vi "test-diff-drive-kine-constraint.vi"(8 "error in (no error)":errorcluster) -> (0 "error out 2":errorcluster, 3 "Test Passed":bool)   [LabVIEW 2019]
uses:
  <vilib>/Rock Robotics/WPI/ThirdParty/JAS_Junk/TrajLib/POSE2D.ctl
  <vilib>/Rock Robotics/WPI/ThirdParty/JAS_Junk/TrajLib/TRANSLATION2D.ctl
  <vilib>/Rock Robotics/WPI/ThirdParty/JAS_Junk/TrajLib/ROTATION2D.ctl
  <vilib>/Rock Robotics/SystemInterfaces/NetworkCommunication/NetComm_UsageReport_report.vi
  <vilib>/Rock Robotics/WPI/ThirdParty/JAS_Junk/TrajLib/DiffDriveKinematicsConstraint_New.vi
  <vilib>/Rock Robotics/WPI/ThirdParty/JAS_Junk/TrajLib/Util_LibraryGlobals.vi
  <vilib>/Rock Robotics/WPI/ThirdParty/JAS_Junk/TrajLib/Trajectory_Library.lvlib
panel:
  out "Accel Exceeded":bool
  out "Acceleration":dbl[][](graph)
  out "Velocity":dbl[][](graph)
  out "Max Accel":dbl
  out "Max Ya":dbl
  out "max Xx":dbl
  in  "Feet/Sec":dbl=12.0 format="%#_13g"
  in  "Feet Per Sec^2":dbl=12.0 format="%#_13g"
  out "Max Speed":dbl
  out "Max Y vel":dbl
  out "max X vel":dbl
  out "XY Graph":cluster{dbl[], dbl[]}[](graph)
  out "Waypoints":T1[](array[typedef]) {"ROTATION"."SIN" format="%13.4f"; "ROTATION"."COS" format="%13.4f"; "ROTATION"."VALUE" format="%13.4f"; "TRANSLATION"."Y" format="%14.3f"; "TRANSLATION"."X" format="%14.3f"}
  out "TotalTImeSecs":dbl
  out "Speed Exceeded":bool
  out "error out":errorcluster
  # "9.1"
  # "5.7"
  # "9.55"
  # "6.59"
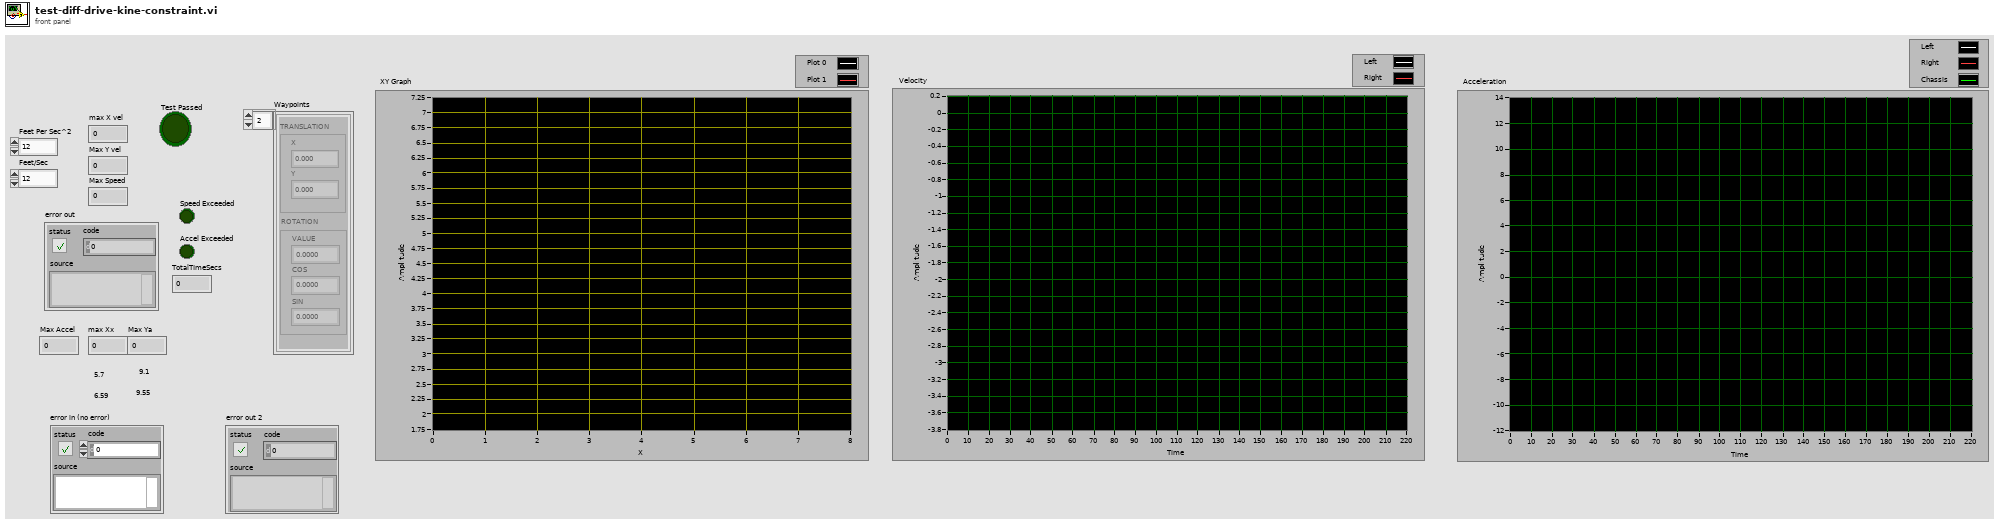
[diagram p1: front panel]
types:
  T1 = typedef "Trajectory_Library.lvlib/POSE2D.ctl" = cluster{"TRANSLATION":T2, "ROTATION":T3}
  T2 = typedef "Trajectory_Library.lvlib/TRANSLATION2D.ctl" = cluster{"X":dbl, "Y":dbl}
  T3 = typedef "Trajectory_Library.lvlib/ROTATION2D.ctl" = cluster{"VALUE":dbl, "COS":dbl, "SIN":dbl}
  T4 = typedef "Trajectory_Library.lvlib/TRAJ_CONFIG.ctl" = cluster{"MaxVelocity":dbl, "Max Acceleration":dbl, "StartVelocity":dbl, "End Velocity":dbl, "Reversed":bool, "DiffDrKineConstntDefined":bool, "CentAcellConstntDefined":bool, "DiffDrVoltConstntDefined":bool, "DIFF_DRIVE_KINE_CONSTRAINT":T5, "CENTRIPETAL_ACCEL_CONSTRAINT":T7, "SwerveDrKineConstntDefined":bool, "SWERVE_DRIVE_KINE_CONSTRAINT":T8, "DIFF_DRIVE_VOLTAGE_CONSTRAINT":T11, "MECANUM_DRIVE_KINE_CONSTRAINT":T13, "MecanumDrKineConstntDefined":bool}
  T5 = typedef "Trajectory_Library.lvlib/TRAJ_CONSTRAINT_DIIF_DRIVE_KINEMATICS.ctl" = cluster{"Max Speed (M/S)":dbl, "DIFF_DRIVE_KINEMATICS":T6, "Max Accel (M/S2)":dbl}
  T6 = typedef "Trajectory_Library.lvlib/DIFF_DRIVE_KINEMATICS.ctl" = cluster{"TrackWidth_Meters":dbl}
  T7 = typedef "Trajectory_Library.lvlib/TRAJ_CONSTRAINT_CENTRIPETAL_ACCEL.ctl" = cluster{"Max Cent Accel":dbl}
  T8 = typedef "Trajectory_Library.lvlib/TRAJ_CONSTRAINT_SWERVE_DRIVE_KINEMATICS.ctl" = cluster{"Max Speed (M/S)":dbl, "SwerveKinematics":T9}
  T9 = typedef "Trajectory_Library.lvlib/SWERVE_DRIVE_KINEMATICS.ctl" = cluster{"NumModules":i32, "InverseKinematics":T10, "ForwardKinematics":T10, "Modules":T2[], "PrevCoR":T2}
  T10 = typedef "NI_Matrix.lvlib/RealMatrix.ctl" = dbl[][]
  T11 = typedef "Trajectory_Library.lvlib/TRAJ_CONSTRAINT_DIIF_DRIVE_VOLTAGE.ctl" = cluster{"Max Voltage":dbl, "DIFF_DRIVE_KINEMATICS":T6, "SIMPLE_MOTOR_FF":T12}
  T12 = typedef "Trajectory_Library.lvlib/SIMPLE_MOTOR_FF.ctl" = cluster{"Ks":dbl, "Kv":dbl, "Ka":dbl}
  T13 = typedef "Trajectory_Library.lvlib/TRAJ_CONSTRAINT_MECA_DRIVE_KINEMATICS.ctl" = cluster{"Max Speed (M/S)":dbl, "MECA_DRIVE_KINEMATICS":T14}
  T14 = typedef "Trajectory_Library.lvlib/MECA_DRIVE_KINEMATICS.ctl" = cluster{"FrontLeft":T2, "FrontRight":T2, "RearLeft":T2, "RearRight":T2, "InverseKinematics":T10, "ForwardKinematics":T10, "PrevCoR":T2}
  T15 = typedef "Trajectory_Library.lvlib/TRAJECTORY.ctl" = cluster{"TotalTImeSecs":dbl, "States":T16[]}
  T16 = typedef "Trajectory_Library.lvlib/TRAJ_STATE.ctl" = cluster{"TimeSeconds":dbl, "Velocity":dbl, "Acceleration":dbl, "POSE":T1, "Curvature":dbl}
  T17 = typedef "Trajectory_Library.lvlib/CHASSIS_SPEEDS.ctl" = cluster{"vX":dbl, "vY":dbl, "vOmega":dbl}
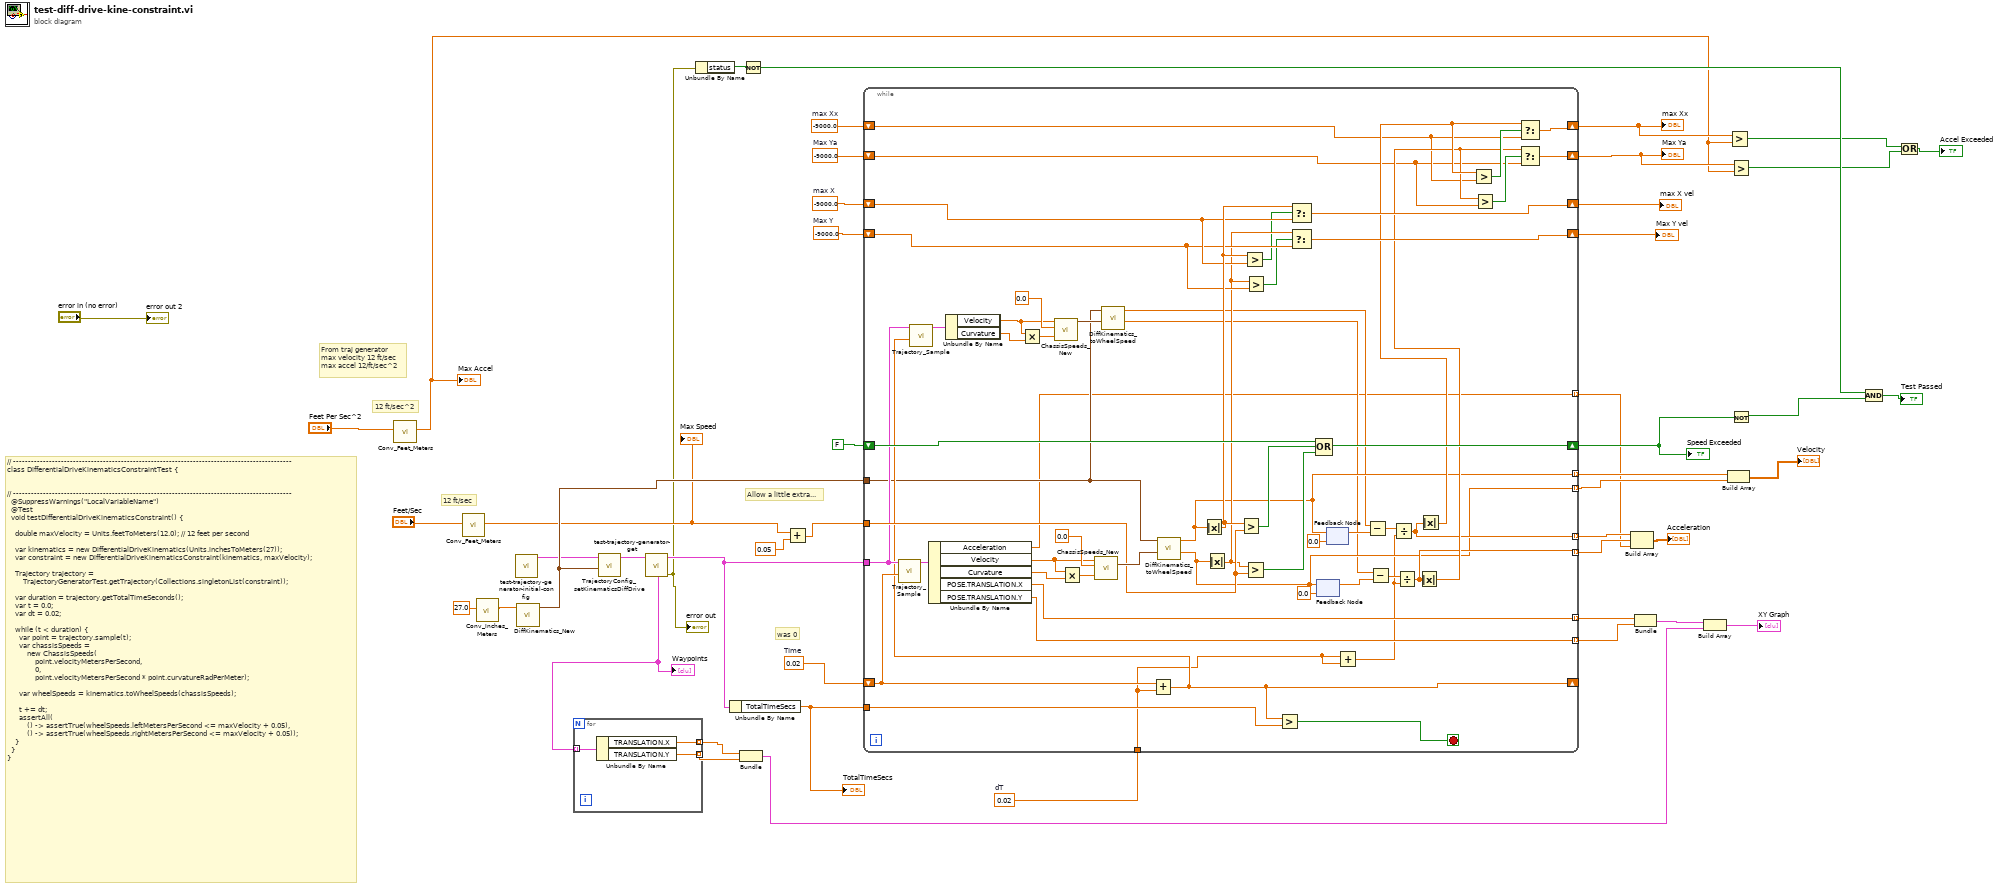
[diagram p0: block diagram]
diagram:
  w17 = -9000.0  # max Xx
  w18 = -9000.0  # Max Ya
  w27 = -9000.0  # max X
  w28 = -9000.0  # Max Y
  w43 = 0.02  # dT
  w45 = 0.02  # TIme
  # "was 0"
  # "Allow a little extra..."
  # "12 ft/sec^2"
  # "From traj generator\nmax velocity 12 ft/sec\nmax accel 12/ft/sec^2"
  # "12 ft/sec"
  # "// ---------------------------------------------------------------------------------------------\nclass DifferentialDriveKinematicsConstraintTest {\n\n\n// ---------------------------------------------------------------------------------------------\n  @SuppressWarnings(\"LocalVariableName\")\n  @Test\n  void testDifferentialDriveKinematicsConstraint() {\n\n    double maxVelocity = Units.feetToMeters(12.0); // 12 feet per second\n\n    var kinematics = new DifferentialDriveKinematics(Units.inchesToMeters(27));\n    var constraint = new DifferentialDriveKinematicsConstraint(kinematics, maxVelocity);\n\n    Trajectory trajectory =\n        TrajectoryGeneratorTest.getTrajectory(Collections.singletonList(constraint));\n\n    var duration = trajectory.getTotalTimeSeconds();\n    var t = 0.0;\n    var dt = 0.02;\n\n    while (t < duration) {\n      var point = trajectory.sample(t);\n      var chassisSpeeds =\n          new ChassisSpeeds(\n              point.velocityMetersPerSecond,\n              0,\n              point.velocityMetersPerSecond * point.curvatureRadPerMeter);\n\n      var wheelSpeeds = kinematics.toWheelSpeeds(chassisSpeeds);\n\n      t += dt;\n      assertAll(\n          () -> assertTrue(wheelSpeeds.leftMetersPerSecond <= maxVelocity + 0.05),\n          () -> assertTrue(wheelSpeeds.rightMetersPerSecond <= maxVelocity + 0.05));\n    }\n  }\n}"
  n1 = call <vilib>:"Conv_Feet_Meters.vi"("Feet"="Feet Per Sec^2") -> ("Meters"=w4:dbl)  [unwired: 10 in]
  "Max Accel" <- w4
  n2 = call <vilib>:"Conv_Feet_Meters.vi"("Feet"="Feet/Sec") -> ("Meters"=w39:dbl)  [unwired: 10 in]
  "Max Speed" <- w39
  n3 = call <vilib>:"Conv_Inches_Meters.vi"("INCH"=27.0) -> ("Meters"=w49:dbl)  [unwired: 10 in]
  n4 = call "test-trajectory-generator-initial-config.vi"() -> ("traj_config"=w2:T4)  [unwired: 11 in]
  n5 = call <vilib>:"DiffKinematics_New.vi"("TrackWidth_Meters"=w49) -> ("DIFF_DRIVE_KINEMATICS"=w41:T6)  [unwired: 10 in]
  n6 = call <vilib>:"TrajectoryConfig_setKinematicsDiffDrive.vi"("DIFF_DRIVE_KINEMATICS"=w41, "inTRAJECTORY_CONFIG"=w2) -> ("outTRAJECTORY_CONFIG"=w3:T4)  [unwired: 9 in]
  n7 = call "test-trajectory-generator-get.vi"("traj_config"=w3) -> ("error out"=w21:errorcluster, "TRAJECTORY"=w42:T15, "Waypoints"=w36:T1[])  [unwired: 8 in]
  "error out" <- w21
  "Waypoints" <- w36
  n8 = for {
    tunnel: w36 -> [w52] mode=indexing
    tunnel: [w51] -> w35 mode=indexing
    tunnel: [w50] -> w34 mode=indexing
    n9 = Unbundle By Name(w52) -> ("TRANSLATION.X"=w51:dbl, "TRANSLATION.Y"=w50:dbl)
  }
  n10 = Unbundle By Name(w21) -> ("status"=w20:bool)
  n11 = Unbundle By Name(w42) -> ("TotalTImeSecs"=w44:dbl)
  "TotalTImeSecs" <- w44
  n12 = Bundle(w35, w34) -> (w30:cluster{dbl[], dbl[]})  [unwired: 1 in]
  n13 = Not(x=w20) -> (.not. x?=w19:bool)
  n14 = Add(x=w39, y=0.05) -> (x+y=w38:dbl)
  n15 = while {
    tunnel: w44 -> [w108]
    shift-right: [w65] -> _
    shift-left: w45 -> [w106]
    tunnel: w43 -> [w54]
    tunnel: w42 -> [w66]
    tunnel: w41 -> [w59]
    shift-right: [w98] -> w22
    shift-left: FALSE -> [w99]
    tunnel: w38 -> [w95]
    tunnel: [w94] -> w33 mode=indexing
    tunnel: [w93] -> w32 mode=indexing
    shift-right: [w91] -> w26
    shift-left: w27 -> [w89]
    shift-right: [w92] -> w25
    shift-left: w28 -> [w88]
    shift-right: [w72] -> w8
    shift-left: w17 -> [w74]
    shift-right: [w71] -> w7
    shift-left: w18 -> [w73]
    tunnel: [w70] -> w16 mode=indexing
    tunnel: [w57] -> w15 mode=indexing
    tunnel: [w69] -> w13 mode=indexing
    tunnel: [w68] -> w12 mode=indexing
    tunnel: [w53] -> w10 mode=indexing
    stop <- w107 stop-if-true
    n16 = call <vilib>:"Trajectory_Sample.vi"("Time"=w106, "InputTRAJECTORY"=w66) -> ("OutputTRAJ_STATE"=w105:T16)  [unwired: 9 in]
    n17 = Unbundle By Name(w105) -> ("Acceleration"=w53:dbl, "Velocity"=w102:dbl, "Curvature"=w101:dbl, "POSE.TRANSLATION.X"=w94:dbl, "POSE.TRANSLATION.Y"=w93:dbl)
    n18 = Multiply(x=w102, y=w101) -> (x*y=w103:dbl)
    n19 = call <vilib>:"ChassisSpeeds_New.vi"("vAngular"=w103, "vY"=0.0, "vX"=w102) -> ("CHASSIS"=w100:T17)  [unwired: 8 in]
    n20 = Add(x=w106, y=w54) -> (x+y=w65:dbl)
    n21 = call <vilib>:"Trajectory_Sample.vi"("Time"=w65, "InputTRAJECTORY"=w66) -> ("OutputTRAJ_STATE"=w67:T16)  [unwired: 9 in]
    n22 = Unbundle By Name(w67) -> ("Velocity"=w62:dbl, "Curvature"=w61:dbl)
    n23 = Multiply(x=w62, y=w61) -> (x*y=w63:dbl)
    n24 = call <vilib>:"ChassisSpeeds_New.vi"("vAngular"=w63, "vY"=0.0, "vX"=w62) -> ("CHASSIS"=w60:T17)  [unwired: 8 in]
    n25 = call <vilib>:"DiffKinematics_toWheelSpeed.vi"("CHASSIS Speed"=w60, "DIFF_DRIVE_KINEMATICS"=w59) -> ("RightVelocity"=w56:dbl, "LeftVelocity"=w58:dbl)  [unwired: 8 in]
    n26 = call <vilib>:"DiffKinematics_toWheelSpeed.vi"("CHASSIS Speed"=w100, "DIFF_DRIVE_KINEMATICS"=w59) -> ("RightVelocity"=w57:dbl, "LeftVelocity"=w70:dbl)  [unwired: 8 in]
    n27 = Absolute Value(x=w70) -> (abs(x)=w90:dbl)
    n28 = Absolute Value(x=w57) -> (abs(x)=w87:dbl)
    n29 = Greater?(x=w90, y=w95) -> (0:w97:bool)
    n30 = Greater?(x=w90, y=w89) -> (0:w86:bool)
    n31 = Greater?(x=w87, y=w95) -> (0:w96:bool)
    n32 = Greater?(x=w87, y=w88) -> (0:w85:bool)
    n33 = Greater?(x=w65, y=w108) -> (0:w107:bool)
    n34 = Select(t=w90, s=w86, f=w89) -> (s? t:f=w91:dbl)
    n35 = Select(t=w87, s=w85, f=w88) -> (s? t:f=w92:dbl)
    n36 = Compound Arithmetic op=OR(w99, w97, w96) -> (w98:bool)
    n37 = feedback #1(0.0 ("RightVelocity")) -> (w81:dbl)
    n38 = feedback-in #1(w57) -> ()
    n39 = feedback-in #2(w70) -> ()
    n40 = feedback #2(0.0 ("LeftVelocity")) -> (w82:dbl)
    n41 = Add(x=w54, y=w54) -> (x+y=w55:dbl)
    n42 = Subtract(x=w58, y=w82) -> (x-y=w80:dbl)
    n43 = Subtract(x=w56, y=w81) -> (x-y=w79:dbl)
    n44 = Divide(x=w80, y=w55) -> (x/y=w69:dbl)
    n45 = Divide(x=w79, y=w55) -> (x/y=w68:dbl)
    n46 = Absolute Value(x=w68) -> (abs(x)=w75:dbl)
    n47 = Absolute Value(x=w69) -> (abs(x)=w76:dbl)
    n48 = Greater?(x=w76, y=w74) -> (0:w78:bool)
    n49 = Greater?(x=w75, y=w73) -> (0:w77:bool)
    n50 = Select(t=w76, s=w78, f=w74) -> (s? t:f=w72:dbl)
    n51 = Select(t=w75, s=w77, f=w73) -> (s? t:f=w71:dbl)
  }
  "Speed Exceeded" <- w22
  "max X vel" <- w26
  "Max Y vel" <- w25
  "max Xx" <- w8
  "Max Ya" <- w7
  n52 = Build Array(w13, w12, w10) -> (→"Acceleration":dbl[][])
  n53 = Bundle(w33, w32) -> (w31:cluster{dbl[], dbl[]})  [unwired: 1 in]
  n54 = Build Array(w31, w30) -> (→"XY Graph":cluster{dbl[], dbl[]}[])
  n55 = Build Array(w16, w15) -> (→"Velocity":dbl[][])
  n56 = Greater?(x=w8, y=w4) -> (0:w6:bool)
  n57 = Greater?(x=w7, y=w4) -> (0:w5:bool)
  n58 = Not(x=w22) -> (.not. x?=w23:bool)
  n59 = Compound Arithmetic op=AND(w19, w23) -> (→"Test Passed":bool)
  n60 = Compound Arithmetic op=OR(w6, w5) -> (→"Accel Exceeded":bool)
  "error out 2" <- "error in (no error)"
